vi "Destroy.vi"(8 "error in (no error)":errorcluster, 11 "Motor Controller in":refnum<class "Motor Controller.lvclass">) -> (0 "error out":errorcluster, 3 "Motor Controller out":refnum<class "Motor Controller.lvclass">)   [LabVIEW 2022 SP3, in "Motor Controller.lvclass"]
uses:
  Motor Controller.lvclass
  Motor Controller.lvclass/Motor Controller.ctl
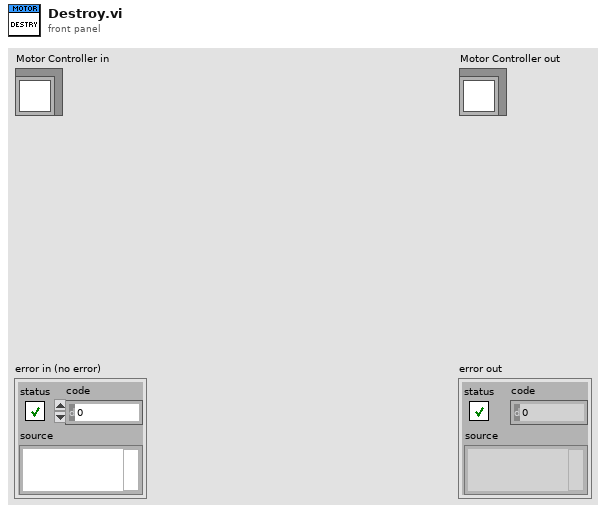
[diagram p1: front panel]
types:
  T1 = typedef "Motor Controller.lvclass/Private Data.ctl" = cluster{"UserEvents":T2, "All Dependencies":cluster{"Class References":refnum<class>[], "Class Names":string[]}, "Status":T3}
  T2 = typedef "Motor Controller.lvclass/UserEvents.ctl" = cluster{"API Incoming Event":refnum<user-event>, "API Executed Event":refnum<user-event>, "API Return Event":refnum<user-event>, "Status Changed Event":refnum<user-event>, "StopEvent":refnum<user-event>}
  T3 = typedef "Motor Controller.lvclass/Status.ctl" = cluster{"Motor Controller Config Data":T4, "Motor Controller Data":cluster{"Enabled?":bool}, "Stage Move":T5, "Stage Busy?":bool}
  T4 = typedef "Motor Controller.lvclass/Motor Controller Config Data.ctl" = cluster{"Motor IP Addresss":string, "Current Position":i32, "Pulse_Per_mm":i32, "PrePrint":dbl[], "Load Position_mm":i32, "Laminate Position_mm":i32}
  T5 = typedef "Motor Controller.lvclass/Stage Move Data.ctl" = cluster{"Current Step":string, "Move Data":T6[]}
  T6 = typedef "Motor Controller.lvclass/Batch Index Speed Data.ctl" = cluster{"Batch & Cycle":string, "Move":cluster{"Index_mm":i32, "Speed_mm_s":i32}, "Status":T7}
  T7 = typedef "Motor Controller.lvclass/Move Status.ctl" = enum16{"Pending", "In Progress", "Completed"}
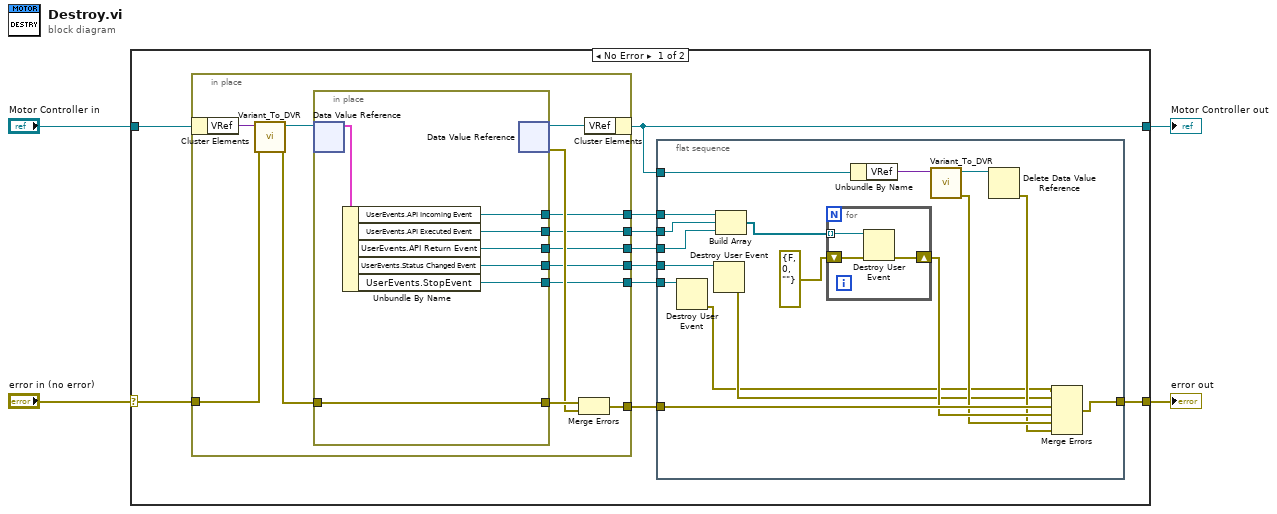
[diagram p0: block diagram]
diagram:
  n1 = case shown="No Error" "error in (no error)" {
    selector: "error in (no error)" -> [w13 w56]
    tunnel: [w9 w56] -> w3
    tunnel: [w10 w55] -> w1
    tunnel: "Motor Controller in" -> [w14 w55]
    frame No Error {
      n2 = in-place {
        in-place-border: w13 -> [w44]
        in-place-border: [w40] -> w11
        in-place-border: [w39] -> w12
        in-place-border: [w38] -> w8
        in-place-border: [w37] -> w7
        in-place-border: [w36] -> w6
        in-place-border: [w35] -> w5
        n3 = in-place-cluster #1(w14) -> ("VRef"=w47:variant)
        n4 = call "Variant_To_DVR.vi"("error in (no error)"=w44, "Variant"=w47) -> ("error out"=w43:errorcluster, "DVR"=w46:refnum<data-value>)  [unwired: 8 in]
        n5 = in-place {
          in-place-border: [w53] -> w39
          in-place-border: w43 -> [w52]
          in-place-border: [w52] -> w42
          in-place-border: [w51] -> w38
          in-place-border: [w50] -> w37
          in-place-border: [w49] -> w36
          in-place-border: [w48] -> w35
          n6 = in-place-dvr #2(w46) -> (w54:T1)  [unwired: 1 out]
          n7 = Unbundle By Name(w54) -> ("UserEvents.API Incoming Event"=w53:refnum<user-event>, "UserEvents.API Executed Event"=w51:refnum<user-event>, "UserEvents.API Return Event"=w50:refnum<user-event>, "UserEvents.Status Changed Event"=w49:refnum<user-event>, "UserEvents.StopEvent"=w48:refnum<user-event>)
          n8 = in-place-dvr #2() -> (w45:refnum<data-value>, w41:errorcluster)  [unwired: 1 in]
        }
        n9 = Merge Errors(w42, w41) -> (w40:errorcluster)
        n10 = in-place-cluster #1("VRef"=w45) -> (w10:refnum<class "Motor Controller.lvclass">)
      }
      n11 = flat-sequence {
        tunnel: w12 -> [w22]
        tunnel: w11 -> [w27]
        tunnel: w10 -> [w30]
        tunnel: [w25] -> w9
        tunnel: w8 -> [w21]
        tunnel: w7 -> [w20]
        tunnel: w6 -> [w18]
        tunnel: w5 -> [w16]
        frame #0 {
          n12 = Destroy User Event(user event=w16) -> (error out=w15:errorcluster)  [unwired: 1 in]
          n13 = Destroy User Event(user event=w18) -> (error out=w17:errorcluster)  [unwired: 1 in]
          n14 = Build Array(w22, w21, w20) -> (w19:refnum<user-event>[])
          n15 = for {
            tunnel: w19 -> [w34] mode=indexing
            shift-right: [w33] -> w26
            shift-left: errorcluster {"status"=FALSE, "code"=0, "source"=""} ("error constant") -> [w32]
            n16 = Destroy User Event(user event=w34, error in=w32) -> (error out=w33:errorcluster)
          }
          n17 = Unbundle By Name(w30) -> ("VRef"=w29:variant)
          n18 = call "Variant_To_DVR.vi"("Variant"=w29) -> ("error out"=w24:errorcluster, "DVR"=w28:refnum<data-value>)  [unwired: 9 in]
          n19 = Delete Data Value Reference(data value reference=w28) -> (error out=w23:errorcluster)  [unwired: 1 in, 1 out]
          n20 = Merge Errors(w15, w17, w27, w26, w24, w23) -> (w25:errorcluster)
        }
      }
    }
    frame Error {
    }
  }
  "error out" <- w3
  "Motor Controller out" <- w1
